vi "BioFeedback16(Intermittent Saving).vi"(7 "Frames Per Second":dbl=30.0, 9 "Start Trial":bool, 11 "End Trial":bool, 12 "Data Directory":path, 13 "File Name":string) -> ()   [LabVIEW 2016]
uses:
  customSubVIs/Control 1.ctl
  <vilib>/Waveform/WDTFileIO.llb/Export Waveforms To Spreadsheet File (1D).vi
  <vilib>/Utility/file.llb/Write Delimited Spreadsheet (DBL).vi
  <vilib>/Utility/file.llb/Write Delimited Spreadsheet (I64).vi
  <vilib>/Utility/error.llb/DialogType.ctl
panel:
  out "MVC Buffer Index":dbl=3.0
  in  "DisplayDataPath":path
  in  "FilteredDataPath":path
  in  "RawDataPath":path
  in  "MVC Number":dbl=1.0
  out "Save MVC":bool
  out "Display Buffer":dbl[][](array[numeric])
  out "Display Buffer Index":dbl=3.0
  out "FilteredTrialData Display Channel":waveform(dbl)(graph)
  out "Raw Trial Data Display Channel":waveform(dbl)(graph)
  out "EndProcessTic":u32
  out "StartProcessTic":u32
  out "EndRecordTic":u32
  out "startRecordTic":u32
  out "Start UI":timestamp
  out "UI Elapsed Time":u32
  out "End UI":timestamp
  out "End Process":timestamp
  out "Start Process":timestamp
  out "End Record":timestamp
  out "Start Record":timestamp
  out "Process Elapsed Time":u32
  out "Record Elapsed Time":u32
  out "FilteredTrialData":waveform(dbl)[](graph)
  out "FilteredAndRectified":waveform(dbl)[](graph) caption="Filtered and Rectified"
  out "FilteredDataArray":waveform(dbl)[](array[waveform])
  in  "DisplayChannel":dbl
  out "DisplayTrialData":T1
  out "DisplayValueByChannel":dbl[](array[numeric])
  out "MVCBufferSize":dbl
  in  "MVC Window Size (s)":dbl=0.5
  out "MVC Buffer":dbl[][](array[numeric])
  out "GetMaxStartTime":timestamp
  in  "SecondsToAcquireMax":dbl=10.0
  out "MVCArray":dbl[](array[numeric])
  out "RawTrialData":waveform(dbl)[](array[waveform])
  in  "UI Ampl Error Path":path=path "C:/Users/Tinggroup/Desktop/VRMuscleActivationVisualizer/VRBiofeedback_v2/assets/BiofeedbackAmplitudeError.txt"
  out "DisplayActivation":dbl
  out "Get MVC":bool
  in  "resetMax":bool
  in  "startGetMax":bool
  in  "Amplitude Error":dbl
  in  "UI Data Path":path=path "C:/Users/Tinggroup/Desktop/VRMuscleActivationVisualizer/VRBiofeedback_v2/assets/LeftEMGData.txt"
  in  "EMG Input Device\nProduct Type":string="USB-6009"
  out "DisplayBarActivation":dbl(slide) caption="Left" max=1.0 scale=0.0..100.0
  out "NormalizedSignal8":dbl[](graph)
  out "NormalizedSignal7":dbl[](graph)
  out "NormalizedSignal6":dbl[](graph)
  out "NormalizedSignal5":dbl[](graph)
  out "NormalizedSignal4":dbl[](graph)
  out "NormalizedSignal3":dbl[](graph)
  out "NormalizedSignal2":dbl[](graph)
  out "NormalizedSignal1":dbl[](graph)
  out "Raw Trial Data Wfm":waveform(dbl)[](graph)
  in  "UI Percent Path":path=path "C:/Users/Tinggroup/Desktop/VRMuscleActivationVisualizer/VRBiofeedback_v2/assets/BiofeedbackTargetPercentage.txt"
  in  "Target Percentage":dbl=10.0
  out "Trial In Progress":bool
  in  "Lower Cut-Off":dbl=20.0
  in  "Upper Cut-Off":dbl=300.0
  out "raw data":dynamicdata(graph)
  out "DisplayBufferSize":dbl
  out "Samples per frame":dbl
  out "Reset":bool=TRUE
  in  "Display Window Size (s)":dbl=0.5
  in  "Sample rate (Hz)":dbl=2000.0
  in  "End Program":bool
  # "Data To Be Saved (Not including Max Data)"
  # "Performance Metrics"
  # "Saving Trial Data"
  # "Small Window"
  # "Scale Max"
  # "Filter and Process Parameters"
  # "MVC Buffer"
  # "Set Target"
  # "Display Parameters"
  # "Changes are made instantly and cause moving average to reset to zero"
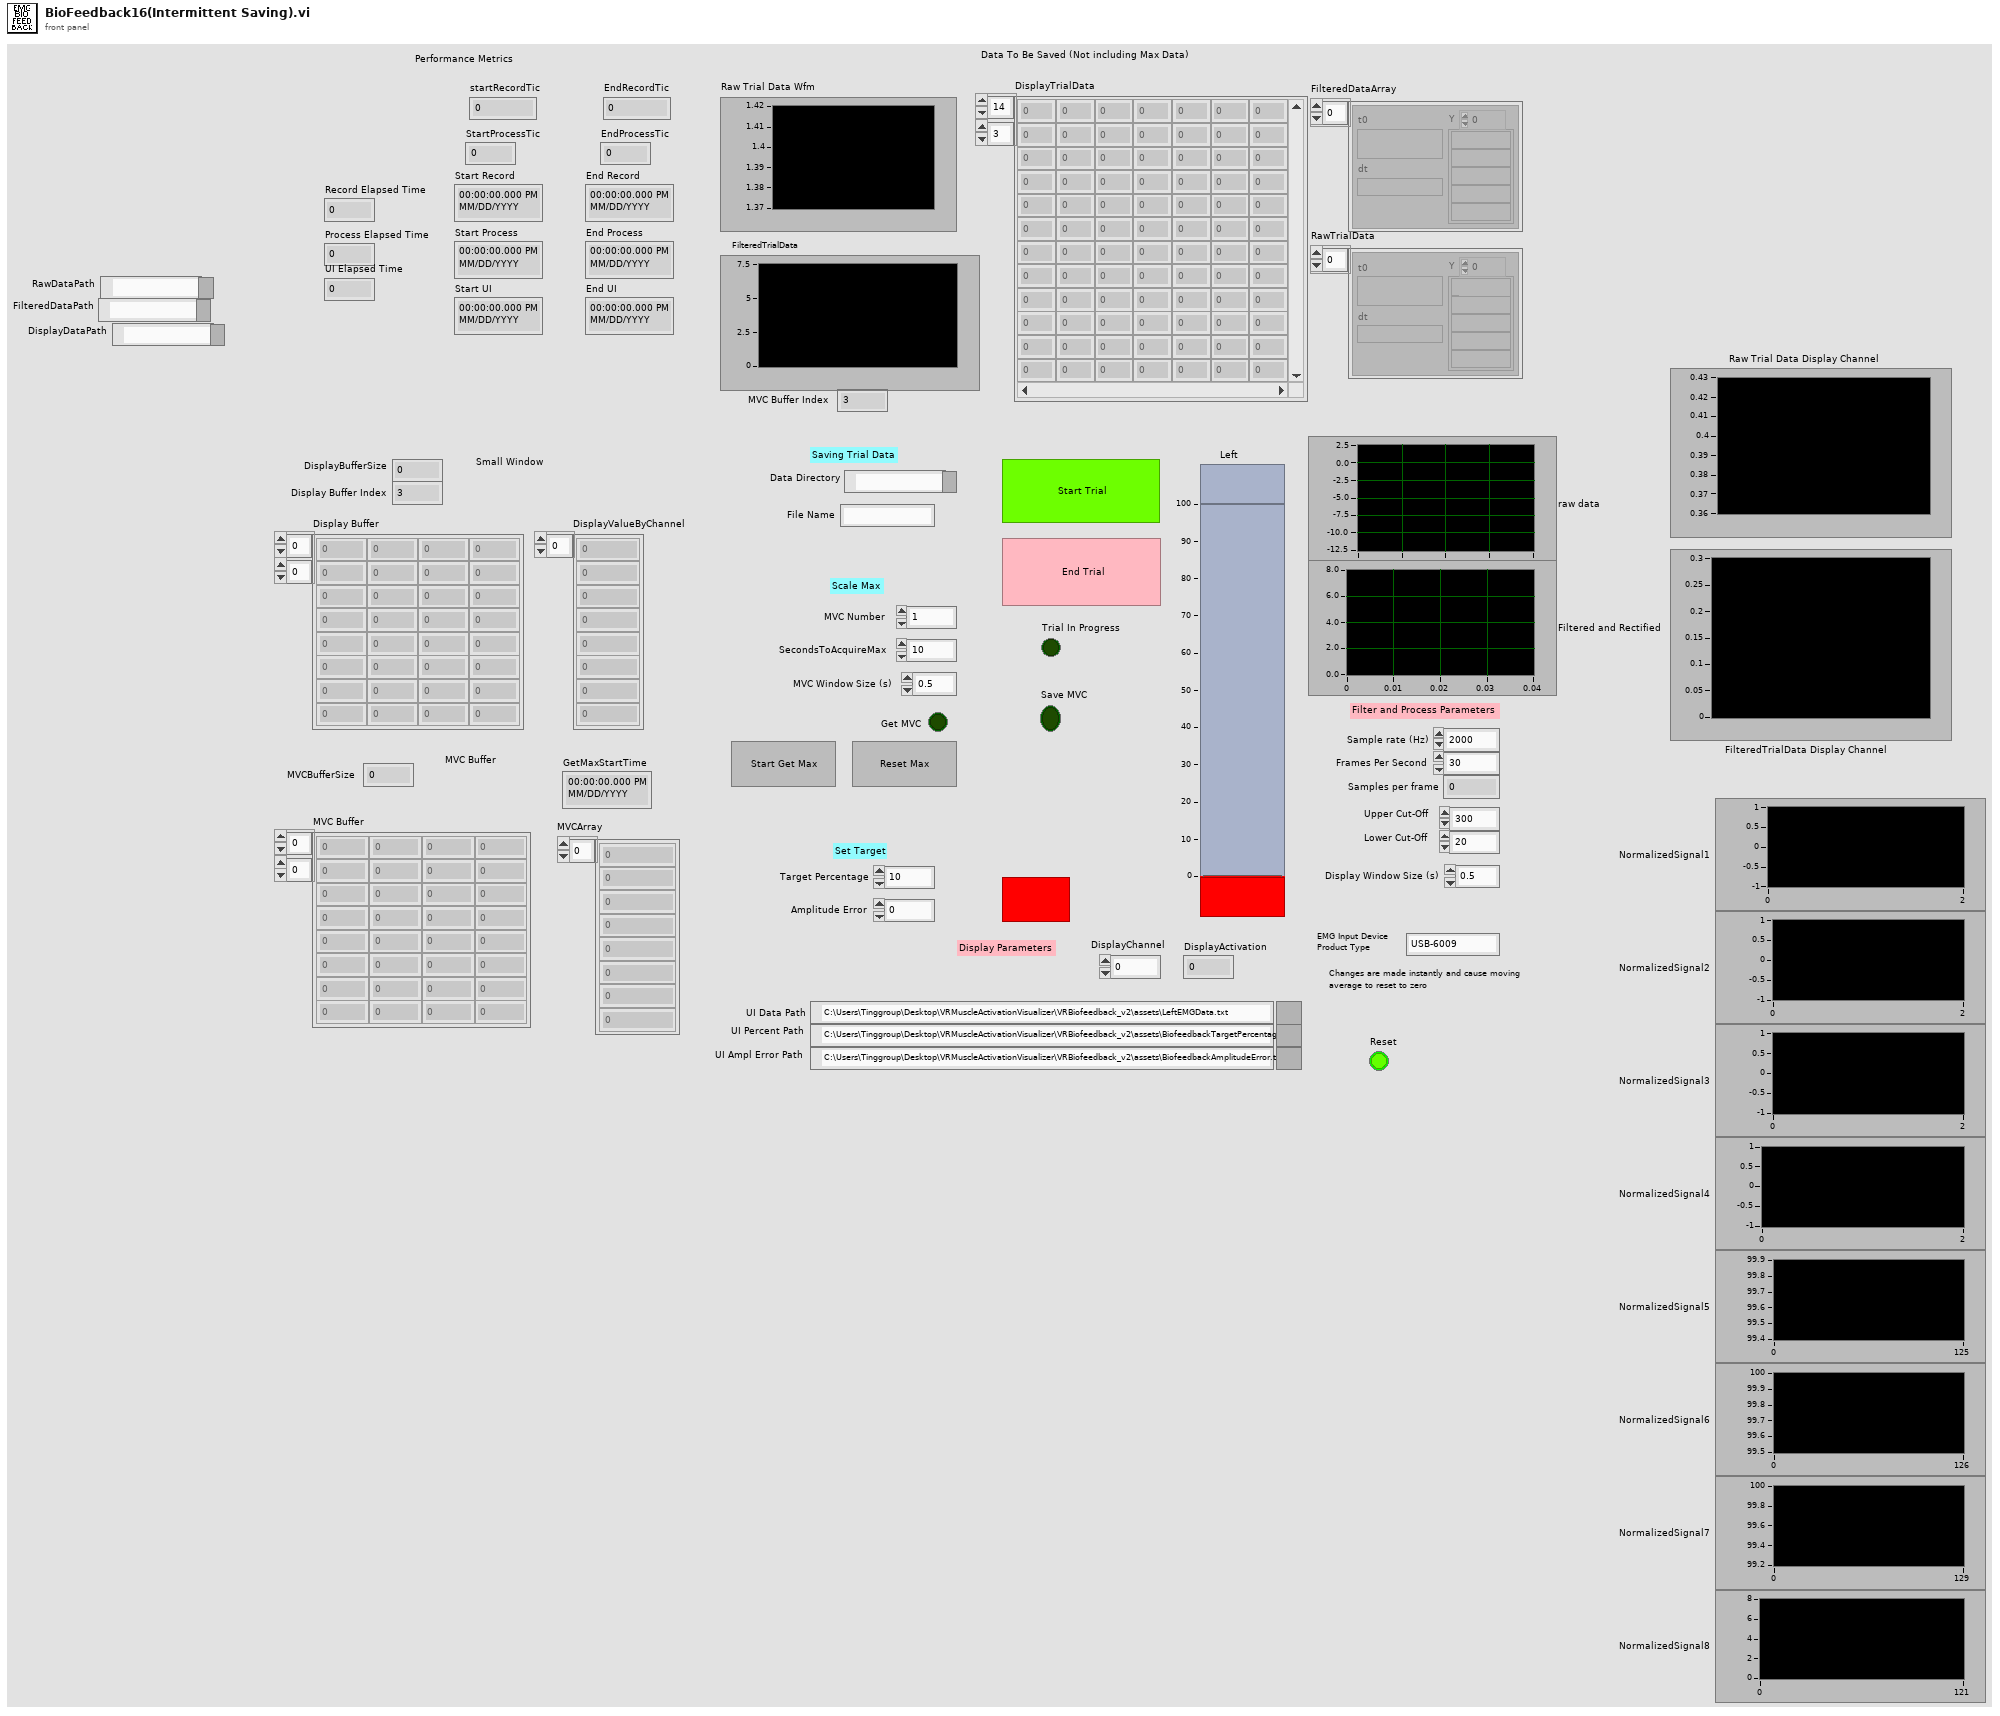
[diagram p1: front panel]
types:
  T1 = typedef "Control 1.ctl" = dbl[][]
  T2 = typedef "DialogType.ctl" = u16
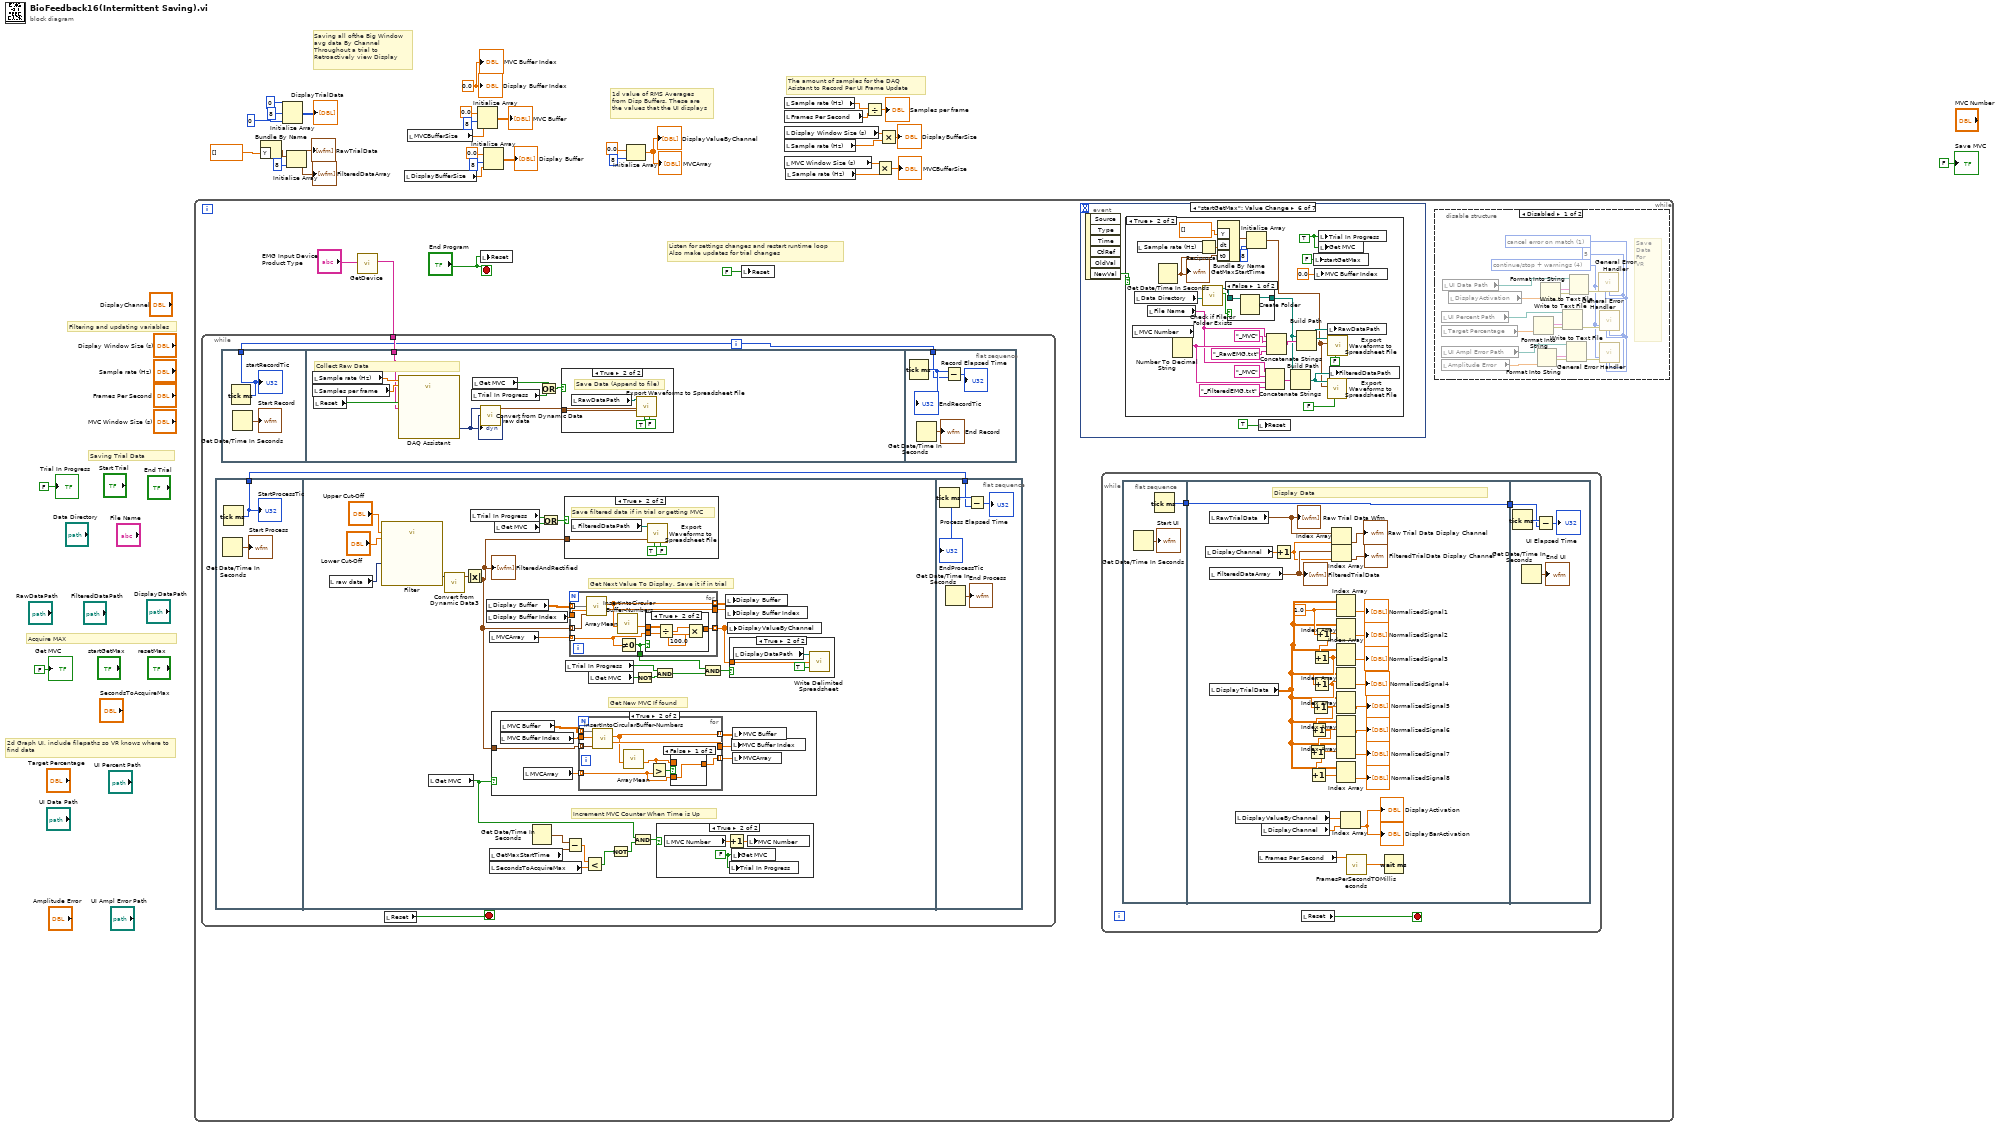
[diagram p0: block diagram]
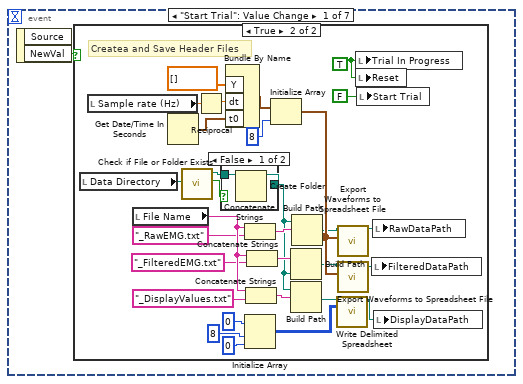
[diagram p3: hidden frame]
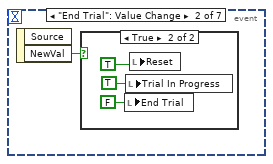
[diagram p6: hidden frame]
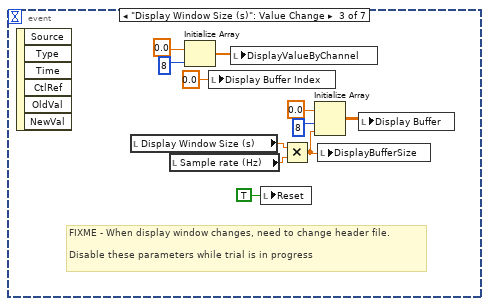
[diagram p8: hidden frame]
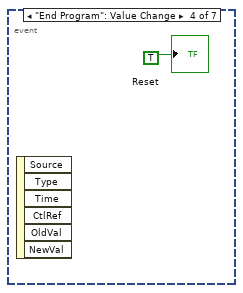
[diagram p9: hidden frame]
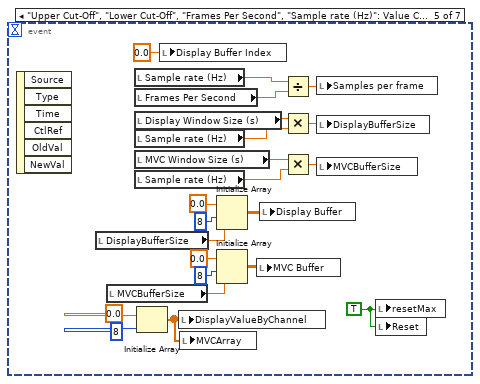
[diagram p10: hidden frame]
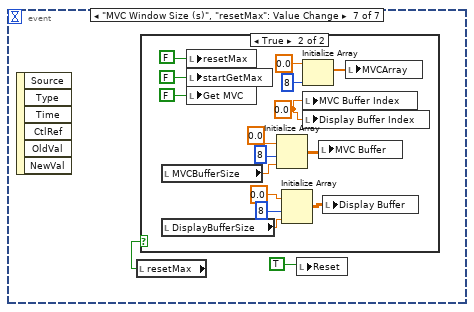
[diagram p13: hidden frame]
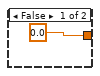
[diagram p19: hidden frame]
diagram:
  w1 = 0.0 ("Display Buffer Index")
  # "The amount of samples for the DAQ Asistant to Record Per UI Frame Update"
  # "Saving all ofthe Big Window \navg data By Channel\nThroughout a trial to \nRetroactively view Display"
  # "1d value of RMS Averages\nfrom Disp Buffers. These are\nthe values that the UI displays"
  # "Acquire MAX"
  # "Filtering and updating variables"
  # "Saving Trial Data"
  # "2d Graph UI, include filepaths so VR knows where to find data"
  n1 = while {
    stop <- "End Program" stop-if-true
    # "Listen for settings changes and restart runtime loop\nAlso make updates for trial changes"
    n2 = call "GetDevice.vi"("EMG Input Device\nProduct Type"="EMG Input Device\nProduct Type") -> ("DAQmx Device Name"=w35:tag)  [unwired: 10 in]
    n3 = while {
      tunnel: w35 -> [w214]
      stop <- w213 stop-if-true
      n4 = flat-sequence {
        tunnel: [w216] -> w212
        tunnel: w212 -> [w290]
        frame #0 {
          n5 = Get Date/Time In Seconds() -> (seconds since 1Jan1904=→"Start Process":timestamp)
          n6 = Tick Count (ms)() -> (millisecond timer value=w216:u32)
          "StartProcessTic" <- w216
        }
        frame #1 {
          # "Increment MVC Counter When Time is Up"
          # "Get New MVC If found"
          # "Get Next Value To Display, Save it if in trial"
          n7 = local read "raw data"() -> (w239:dynamicdata)
          n8 = call "Filter"("Lower Cut-Off"="Lower Cut-Off", "Upper Cut-Off"="Upper Cut-Off", "Signal"=w239) -> ("Filtered Signal"=w245:dynamicdata)  [unwired: 7 in, 1 out]
          n9 = local read "Get MVC"() -> (w223:bool)
          n10 = call "Convert from Dynamic Data3"("Dynamic Data Type"=w245) -> ("Array of Waveform"=w244:waveform(dbl)[])  [unwired: 3 in]
          n11 = Absolute Value(x=w244) -> (abs(x)=w228:waveform(dbl)[])
          "FilteredAndRectified" <- w228
          n12 = local read "Trial In Progress"() -> (w241:bool)
          n13 = local read "Display Buffer"() -> (w237:dbl[][])
          n14 = local read "Display Buffer Index"() -> (w236:dbl)
          n15 = local read "MVCArray"() -> (w233:dbl[])
          n16 = local read "GetMaxStartTime"() -> (w229:timestamp)
          n17 = local read "SecondsToAcquireMax"() -> (w232:dbl)
          n18 = case shown="True" w223 {
            tunnel: w228 -> [_ w256]
            frame False {
            }
            frame True {
              n19 = local read "MVC Buffer Index"() -> (w258:dbl)
              n20 = local read "MVC Buffer"() -> (w257:dbl[][])
              n21 = local read "MVCArray"() -> (w255:dbl[])
              n22 = for {
                tunnel: w257 -> [w267] mode=indexing
                tunnel: w258 -> [w259]
                tunnel: [w266] -> w252
                tunnel: w256 -> [w265] mode=indexing
                tunnel: w255 -> [w261] mode=indexing
                tunnel: [w260] -> w254 mode=indexing
                tunnel: [w262] -> w253 mode=indexing
                n23 = call "InsertIntoCircularBuffer-Numbers.vi"("NewElements"=w265, "StartIndex"=w259, "Buffer"=w267) -> ("New Start Index"=w266:dbl, "UpdatedBuffer"=w262:dbl[])  [unwired: 7 in]
                n24 = call "ArrayMean.vi"("Array"=w262) -> ("Mean"=w263:dbl)  [unwired: 10 in]
                n25 = Greater?(x=w263, y=w261) -> (0:w264:bool)
                n26 = case shown="False" w264 {
                  tunnel: w263 -> [_ w269]
                  tunnel: [w268 w269] -> w260
                  tunnel: w261 -> [w268 _]
                  frame False {
                  }
                  frame True {
                  }
                }
              }
              n27 = local write "MVC Buffer Index"(w252) -> ()
              n28 = local write "MVC Buffer"(w253) -> ()
              n29 = local write "MVCArray"(w254) -> ()
            }
          }
          n30 = local read "Get MVC"() -> (w238:bool)
          n31 = Get Date/Time In Seconds() -> (seconds since 1Jan1904=w230:timestamp)
          n32 = Or(x=w241, y=w238) -> (x .or. y?=w240:bool)
          n33 = case shown="True" w240 {
            tunnel: w228 -> [_ w285]
            frame False {
            }
            frame True {
              # "Save filtered data if in trial or getting MVC"
              n34 = local read "FilteredDataPath"() -> (w286:path)
              n35 = call-poly <vilib>:"Export Waveforms to Spreadsheet File.vi"("header? (write header:T)"=FALSE, "append to file? (new file:F)"=TRUE, "waveforms"=w285, "file path (dialog if empty)"=w286) -> ()  [unwired: 6 in, 2 out]
            }
          }
          n36 = local read "Trial In Progress"() -> (w218:bool)
          n37 = Subtract(x=w230, y=w229) -> (x-y=w231:dbl)
          n38 = for {
            tunnel: w237 -> [w278] mode=indexing
            tunnel: w228 -> [w271] mode=indexing
            tunnel: w236 -> [w277]
            tunnel: [w275] -> w235 mode=indexing
            tunnel: [w276] -> w234
            tunnel: w233 -> [w273] mode=indexing
            tunnel: [w272] -> w224 mode=indexing
            tunnel: [w270] -> w221
            n39 = call "InsertIntoCircularBuffer-Numbers.vi"("NewElements"=w271, "StartIndex"=w277, "Buffer"=w278) -> ("New Start Index"=w276:dbl, "UpdatedBuffer"=w275:dbl[])  [unwired: 7 in]
            n40 = call "ArrayMean.vi"("Array"=w275) -> ("Mean"=w274:dbl)  [unwired: 10 in]
            n41 = Not Equal To 0?(x=w273) -> (x != 0?=w270:bool)
            n42 = case shown="True" w270 {
              tunnel: w274 -> [_ w283]
              tunnel: w273 -> [_ w284]
              tunnel: [0.0 w282] -> w272
              frame False {
              }
              frame True {
                n43 = Divide(x=w283, y=w284) -> (x/y=w281:dbl)
                n44 = Multiply(x=w281, y=100.0) -> (x*y=w282:dbl)
              }
            }
          }
          n45 = Less?(x=w231, y=w232) -> (x < y?=w227:bool)
          n46 = local read "Get MVC"() -> (w220:bool)
          n47 = Not(x=w227) -> (.not. x?=w226:bool)
          n48 = And(x=w223, y=w226) -> (x .and. y?=w225:bool)
          n49 = Not(x=w220) -> (.not. x?=w219:bool)
          n50 = And(x=w218, y=w219) -> (x .and. y?=w217:bool)
          n51 = case shown="True" w225 {
            frame False {
            }
            frame True {
              w249 = FALSE ("Get MVC")
              n52 = local read "MVC Number"() -> (w250:dbl)
              n53 = Increment(x=w250) -> (x+1=w251:dbl)
              n54 = local write "Trial In Progress"(w249) -> ()
              n55 = local write "Get MVC"(w249) -> ()
              n56 = local write "MVC Number"(w251) -> ()
            }
          }
          n57 = And(x=w221, y=w217) -> (x .and. y?=w222:bool)
          n58 = local write "Display Buffer"(w235) -> ()
          n59 = local write "Display Buffer Index"(w234) -> ()
          n60 = local write "DisplayValueByChannel"(w224) -> ()
          n61 = case shown="True" w222 {
            tunnel: w224 -> [_ w247]
            frame False {
            }
            frame True {
              n62 = local read "DisplayDataPath"() -> (w246:path)
              n63 = call-poly <vilib>:"Write Delimited Spreadsheet.vi"("file path (dialog if empty)"=w246, "1D data"=w247, "append to file? (new file:F)"=TRUE) -> ()  [unwired: 11 in, 2 out]
            }
          }
        }
        frame #2 {
          n64 = Tick Count (ms)() -> (millisecond timer value=w291:u32)
          "EndProcessTic" <- w291
          n65 = Get Date/Time In Seconds() -> (seconds since 1Jan1904=→"End Process":timestamp)
          n66 = Subtract(x=w291, y=w290) -> (x-y=→"Process Elapsed Time":u32)
        }
      }
      n67 = flat-sequence {
        tunnel: [w294] -> w211
        tunnel: w214 -> [w299]
        tunnel: w211 -> [w308]
        frame #0 {
          n68 = Tick Count (ms)() -> (millisecond timer value=w294:u32)
          "startRecordTic" <- w294
          n69 = Get Date/Time In Seconds() -> (seconds since 1Jan1904=→"Start Record":timestamp)
        }
        frame #1 {
          # "Collect Raw Data"
          n70 = local read "Sample rate (Hz)"() -> (w302:dbl)
          n71 = local read "Samples per frame"() -> (w301:dbl)
          n72 = local read "Reset"() -> (w300:bool)
          n73 = call "DAQ Assistant"("rate"=w302, "number of samples"=w301, "stop (T)"=w300, "device name"=w299) -> ("data"=w296:dynamicdata)  [unwired: 13 in, 2 out]
          "raw data" <- w296
          n74 = local read "Trial In Progress"() -> (w298:bool)
          n75 = local read "Get MVC"() -> (w297:bool)
          n76 = call "Convert from Dynamic Data"("Dynamic Data Type"=w296) -> ("Array of Waveform"=w303:waveform(dbl)[])  [unwired: 3 in]
          n77 = Or(x=w297, y=w298) -> (x .or. y?=w295:bool)
          n78 = case shown="True" w295 {
            tunnel: w303 -> [_ w305]
            frame False {
            }
            frame True {
              # "Save Data (Append to file)"
              n79 = local read "RawDataPath"() -> (w304:path)
              n80 = call-poly <vilib>:"Export Waveforms to Spreadsheet File.vi"("header? (write header:T)"=FALSE, "append to file? (new file:F)"=TRUE, "waveforms"=w305, "file path (dialog if empty)"=w304) -> ()  [unwired: 6 in, 2 out]
            }
          }
        }
        frame #2 {
          n81 = Tick Count (ms)() -> (millisecond timer value=w309:u32)
          "EndRecordTic" <- w309
          n82 = Get Date/Time In Seconds() -> (seconds since 1Jan1904=→"End Record":timestamp)
          n83 = Subtract(x=w309, y=w308) -> (x-y=→"Record Elapsed Time":u32)
        }
      }
      n84 = local read "Reset"() -> (w213:bool)
    }
    n85 = local write "Reset"("End Program") -> ()
    n86 = local write "Reset"(FALSE) -> ()
    n87 = event shown="[5] \"startGetMax\": Value Change" {
      selector: _ -> [_ _ _ _ _ _ _]
      dyn-events: _ -> [_ _ _ _ _ _ _]
      timeout: _ -> [_ _ _ _ _ _ _]
      event "Start Trial": Value Change {
        n88 = event-data() -> ("NewVal"=w93:bool)  [unwired: 1 in, 1 out]
        n89 = case shown="True" w93 {
          frame False {
          }
          frame True {
            w120 = TRUE ("Trial In Progress")
            # "Createa and Save Header Files"
            n90 = local read "Data Directory"() -> (w107:path)
            n91 = local read "Sample rate (Hz)"() -> (w116:dbl)
            n92 = local read "File Name"() -> (w113:string)
            n93 = Get Date/Time In Seconds() -> (seconds since 1Jan1904=w114:timestamp)
            n94 = call <vilib>:"Check if File or Folder Exists.vi"("path"=w107) -> ("file or folder exists?"=w106:bool, "dup path"=w105:path)  [unwired: 8 in, 1 out]
            n95 = Reciprocal(x=w116) -> (1/x=w115:dbl)
            n96 = case shown="False" w106 {
              tunnel: [w121 w123] -> w104
              tunnel: w105 -> [w122 w123]
              frame False {
                n97 = Create Folder(path (use dialog)=w122) -> (created path=w121:path)  [unwired: 2 in, 2 out]
              }
              frame True {
              }
            }
            n98 = Bundle By Name("Y"=dbl[] [], "dt"=w115, "t0"=w114) -> (w119:waveform(dbl))  [unwired: 1 in]
            n99 = Concatenate Strings(w113, "_RawEMG.txt" ("string")) -> (w108:string)
            n100 = Initialize Array(0, 8 ("dimension size"), 0 ("dimension size")) -> (w95:i32[][])
            n101 = Concatenate Strings(w113, "_DisplayValues.txt" ("string")) -> (w111:string)
            n102 = Concatenate Strings(w113, "_FilteredEMG.txt" ("string")) -> (w109:string)
            n103 = Initialize Array(w119, 8 ("dimension size")) -> (w103:waveform(dbl)[])
            n104 = Build Path(base path=w104, name or relative path=w109) -> (appended path=w100:path)
            n105 = Build Path(base path=w104, name or relative path=w111) -> (appended path=w99:path)
            n106 = Build Path(base path=w104, name or relative path=w108) -> (appended path=w101:path)
            n107 = call-poly <vilib>:"Write Delimited Spreadsheet.vi"("file path (dialog if empty)"=w99, "2D data"=w95) -> ()  [unwired: 12 in, 2 out]
            n108 = call-poly <vilib>:"Export Waveforms to Spreadsheet File.vi"("waveforms"=w103, "file path (dialog if empty)"=w101) -> ()  [unwired: 8 in, 2 out]
            n109 = call-poly <vilib>:"Export Waveforms to Spreadsheet File.vi"("waveforms"=w103, "file path (dialog if empty)"=w100) -> ()  [unwired: 8 in, 2 out]
            n110 = local write "Trial In Progress"(w120) -> ()
            n111 = local write "Reset"(w120) -> ()
            n112 = local write "Start Trial"(FALSE ("Start Trial")) -> ()
            n113 = local write "FilteredDataPath"(w100) -> ()
            n114 = local write "RawDataPath"(w101) -> ()
            n115 = local write "DisplayDataPath"(w99) -> ()
          }
        }
      }
      event "End Trial": Value Change {
        n116 = event-data() -> ("NewVal"=w124:bool)  [unwired: 1 in, 1 out]
        n117 = case shown="True" w124 {
          frame False {
          }
          frame True {
            n118 = local write "End Trial"(FALSE ("End Trial")) -> ()
            n119 = local write "Trial In Progress"(TRUE ("Trial In Progress")) -> ()
            n120 = local write "Reset"(TRUE ("Reset Data Acquisition\nAnd UI Updating")) -> ()
          }
        }
      }
      event "Display Window Size (s)": Value Change {
        # "FIXME - When display window changes, need to change header file.\n\nDisable these parameters while trial is in progress"
        n121 = event-data() -> ()  [unwired: 1 in, 6 out]
        n122 = local read "Display Window Size (s)"() -> (w130:dbl)
        n123 = local read "Sample rate (Hz)"() -> (w129:dbl)
        n124 = Initialize Array(0.0 ("element"), 8 ("dimension size")) -> (w135:dbl[])
        n125 = local write "Display Buffer Index"(0.0 ("Display Buffer Index")) -> ()
        n126 = local write "DisplayValueByChannel"(w135) -> ()
        n127 = local write "Reset"(TRUE ("Reset")) -> ()
        n128 = Multiply(x=w130, y=w129) -> (x*y=w128:dbl)
        n129 = Initialize Array(0.0 ("element"), 8 ("dimension size"), w128) -> (w131:dbl[][])
        n130 = local write "DisplayBufferSize"(w128) -> ()
        n131 = local write "Display Buffer"(w131) -> ()
      }
      event "End Program": Value Change {
        n132 = event-data() -> ()  [unwired: 1 in, 6 out]
        "Reset" <- TRUE
      }
      event "Upper Cut-Off", "Lower Cut-Off", "Frames Per Second", "Sample rate (Hz)": Value Change {
        w146 = TRUE
        n133 = event-data() -> ()  [unwired: 1 in, 6 out]
        n134 = local read "DisplayBufferSize"() -> (w151:dbl)
        n135 = local read "MVCBufferSize"() -> (w143:dbl)
        n136 = local read "Sample rate (Hz)"() -> (w161:dbl)
        n137 = local read "Frames Per Second"() -> (w160:dbl)
        n138 = local read "Display Window Size (s)"() -> (w158:dbl)
        n139 = local read "Sample rate (Hz)"() -> (w157:dbl)
        n140 = local read "MVC Window Size (s)"() -> (w156:dbl)
        n141 = local read "Sample rate (Hz)"() -> (w155:dbl)
        n142 = Initialize Array(0.0 ("element"), 8 ("dimension size")) -> (w145:dbl[])
        n143 = local write "Display Buffer Index"(0.0 ("Display Buffer Index")) -> ()
        n144 = local write "DisplayValueByChannel"(w145) -> ()
        n145 = local write "MVCArray"(w145) -> ()
        n146 = Initialize Array(0.0 ("element"), 8 ("dimension size"), w151) -> (w149:dbl[][])
        n147 = Initialize Array(0.0 ("element"), 8 ("dimension size"), w143) -> (w141:dbl[][])
        n148 = local write "MVC Buffer"(w141) -> ()
        n149 = local write "Display Buffer"(w149) -> ()
        n150 = Divide(x=w161, y=w160) -> (x/y=w159:dbl)
        n151 = Multiply(x=w158, y=w157) -> (x*y=w153:dbl)
        n152 = Multiply(x=w156, y=w155) -> (x*y=w154:dbl)
        n153 = local write "Samples per frame"(w159) -> ()
        n154 = local write "DisplayBufferSize"(w153) -> ()
        n155 = local write "MVCBufferSize"(w154) -> ()
        n156 = local write "resetMax"(w146) -> ()
        n157 = local write "Reset"(w146) -> ()
      }
      event "startGetMax": Value Change {
        n158 = event-data() -> ("NewVal"=w163:bool)  [unwired: 1 in, 5 out]
        n159 = case shown="True" w163 {
          frame False {
          }
          frame True {
            w168 = TRUE ("Trial In Progress")
            n160 = local read "MVC Number"() -> (w182:dbl)
            n161 = local read "Data Directory"() -> (w186:path)
            n162 = local read "Sample rate (Hz)"() -> (w178:dbl)
            n163 = local read "File Name"() -> (w175:string)
            n164 = Get Date/Time In Seconds() -> (seconds since 1Jan1904=w176:timestamp)
            "GetMaxStartTime" <- w176
            n165 = Number To Decimal String(number=w182) -> (decimal integer string=w185:string)  [unwired: 1 in]
            n166 = Reciprocal(x=w178) -> (1/x=w177:dbl)
            n167 = call <vilib>:"Check if File or Folder Exists.vi"("path"=w186) -> ("file or folder exists?"=w183:bool, "dup path"=w190:path)  [unwired: 8 in, 1 out]
            n168 = Bundle By Name("Y"=dbl[] [], "dt"=w177, "t0"=w176) -> (w180:waveform(dbl))  [unwired: 1 in]
            n169 = case shown="False" w183 {
              tunnel: w190 -> [w192 w193]
              tunnel: [w191 w193] -> w172
              frame False {
                n170 = Create Folder(path (use dialog)=w192) -> (created path=w191:path)  [unwired: 2 in, 2 out]
              }
              frame True {
              }
            }
            n171 = Initialize Array(w180, 8 ("dimension size")) -> (w167:waveform(dbl)[])
            n172 = Concatenate Strings(w175, "_MVC" ("string"), w185, "_FilteredEMG.txt" ("string")) -> (w188:string)
            n173 = Concatenate Strings(w175, "_MVC" ("string"), w185, "_RawEMG.txt" ("string")) -> (w187:string)
            n174 = Build Path(base path=w172, name or relative path=w188) -> (appended path=w170:path)
            n175 = Build Path(base path=w172, name or relative path=w187) -> (appended path=w181:path)
            n176 = local write "startGetMax"(FALSE ("Start Trial")) -> ()
            n177 = local write "MVC Buffer Index"(0.0 ("MVC Buffer Indes")) -> ()
            n178 = local write "Trial In Progress"(w168) -> ()
            n179 = local write "Get MVC"(w168) -> ()
            n180 = local write "RawDataPath"(w181) -> ()
            n181 = call-poly <vilib>:"Export Waveforms to Spreadsheet File.vi"("append to file? (new file:F)"=FALSE, "waveforms"=w167, "file path (dialog if empty)"=w170) -> ()  [unwired: 7 in, 2 out]
            n182 = call-poly <vilib>:"Export Waveforms to Spreadsheet File.vi"("append to file? (new file:F)"=FALSE, "waveforms"=w167, "file path (dialog if empty)"=w181) -> ()  [unwired: 7 in, 2 out]
            n183 = local write "FilteredDataPath"(w170) -> ()
          }
        }
        n184 = local write "Reset"(TRUE ("Reset Data Acquisition\nAnd UI Updating")) -> ()
      }
      event "MVC Window Size (s)", "resetMax": Value Change {
        n185 = event-data() -> ()  [unwired: 1 in, 6 out]
        n186 = local read "resetMax"() -> (w194:bool)
        n187 = case shown="True" w194 {
          frame False {
          }
          frame True {
            w196 = 0.0 ("MVC Buffer Index")
            n188 = local read "MVCBufferSize"() -> (w202:dbl)
            n189 = local read "DisplayBufferSize"() -> (w198:dbl)
            n190 = local write "resetMax"(FALSE ("endGetMax")) -> ()
            n191 = local write "startGetMax"(FALSE ("startGetMax")) -> ()
            n192 = local write "Get MVC"(FALSE ("Acquiring Max")) -> ()
            n193 = Initialize Array(0.0 ("element"), 8 ("dimension size"), w202) -> (w201:dbl[][])
            n194 = Initialize Array(0.0 ("element"), 8 ("dimension size"), w198) -> (w197:dbl[][])
            n195 = Initialize Array(0.0 ("element"), 8 ("dimension size")) -> (w205:dbl[])
            n196 = local write "MVC Buffer Index"(w196) -> ()
            n197 = local write "Display Buffer Index"(w196) -> ()
            n198 = local write "MVC Buffer"(w201) -> ()
            n199 = local write "Display Buffer"(w197) -> ()
            n200 = local write "MVCArray"(w205) -> ()
          }
        }
        n201 = local write "Reset"(TRUE ("Reset Data Acquisition\nAnd UI Updating")) -> ()
      }
    }
    n202 = while {
      stop <- w55 stop-if-true
      n203 = flat-sequence {
        tunnel: [w59] -> w57
        tunnel: [w88] -> w56
        tunnel: w57 -> [w88]
        tunnel: w56 -> [w89]
        frame #0 {
          n204 = Get Date/Time In Seconds() -> (seconds since 1Jan1904=→"Start UI":timestamp)
          n205 = Tick Count (ms)() -> (millisecond timer value=w59:u32)
        }
        frame #1 {
          w62 = 1.0 ("x")
          # "Display Data"
          n206 = local read "DisplayChannel"() -> (w83:dbl)
          n207 = local read "RawTrialData"() -> (w78:waveform(dbl)[])
          "Raw Trial Data Wfm" <- w78
          n208 = local read "DisplayTrialData"() -> (w61:T1)
          n209 = local read "FilteredDataArray"() -> (w82:waveform(dbl)[])
          "FilteredTrialData" <- w82
          n210 = local read "DisplayValueByChannel"() -> (w87:dbl[])
          n211 = local read "Frames Per Second"() -> (w85:dbl)
          n212 = local read "DisplayChannel"() -> (w84:dbl)
          n213 = Increment(x=w83) -> (x+1=w81:dbl)
          n214 = Increment(x=w62) -> (x+1=w63:dbl)
          n215 = Increment(x=w63) -> (x+1=w64:dbl)
          n216 = Increment(x=w64) -> (x+1=w65:dbl)
          n217 = Increment(x=w65) -> (x+1=w66:dbl)
          n218 = Increment(x=w66) -> (x+1=w67:dbl)
          n219 = Increment(x=w67) -> (x+1=w68:dbl)
          n220 = Increment(x=w68) -> (x+1=w69:dbl)
          n221 = Index Array(array=w78, index=w81) -> (element=→"Raw Trial Data Display Channel":waveform(dbl))
          n222 = Index Array(array=w82, index=w81) -> (element=→"FilteredTrialData Display Channel":waveform(dbl))
          n223 = Index Array(array=w61, index (row)=w62) -> (element=→"NormalizedSignal1":dbl[])  [unwired: 1 in]
          n224 = Index Array(array=w61, index (row)=w63) -> (element=→"NormalizedSignal2":dbl[])  [unwired: 1 in]
          n225 = Index Array(array=w61, index (row)=w64) -> (element=→"NormalizedSignal3":dbl[])  [unwired: 1 in]
          n226 = Index Array(array=w61, index (row)=w65) -> (element=→"NormalizedSignal4":dbl[])  [unwired: 1 in]
          n227 = Index Array(array=w61, index (row)=w66) -> (element=→"NormalizedSignal5":dbl[])  [unwired: 1 in]
          n228 = Index Array(array=w61, index (row)=w67) -> (element=→"NormalizedSignal6":dbl[])  [unwired: 1 in]
          n229 = Index Array(array=w61, index (row)=w68) -> (element=→"NormalizedSignal7":dbl[])  [unwired: 1 in]
          n230 = Index Array(array=w61, index (row)=w69) -> (element=→"NormalizedSignal8":dbl[])  [unwired: 1 in]
          n231 = Index Array(array=w87, index=w84) -> (element=→"DisplayBarActivation" →"DisplayActivation":dbl)
          n232 = call "FramesPerSecondTOMilliseconds.vi"("Thermometer\nFps"=w85) -> ("x*y"=w86:dbl)  [unwired: 10 in]
          n233 = Wait (ms)(milliseconds to wait=w86) -> ()  [unwired: 1 out]
        }
        frame #2 {
          n234 = Tick Count (ms)() -> (millisecond timer value=w90:u32)
          n235 = Get Date/Time In Seconds() -> (seconds since 1Jan1904=→"End UI":timestamp)
          n236 = Subtract(x=w90, y=w89) -> (x-y=→"UI Elapsed Time":u32)
        }
      }
      n237 = local read "Reset"() -> (w55:bool)
    }
    n238 = disable-structure shown="Disabled" {
      frame Disabled {
        w39 = T2 4 items=["no dialog", "OK message", "continue or stop message", "OK message + warnings", "continue/stop + warnings"] ("type of dialog (OK msg:1)")
        w38 = 1 items=["no exception", "cancel error on match", "set error on match"] ("[exception action] (none:0)")
        w37 = 5 ("[exception code]")
        # "Save\nData\nFor\nVR"
        n239 = local read "UI Ampl Error Path"() -> (w40:path)
        n240 = local read "Amplitude Error"() -> (w41:dbl)
        n241 = local read "UI Percent Path"() -> (w46:path)
        n242 = local read "Target Percentage"() -> (w45:dbl)
        n243 = local read "UI Data Path"() -> (w52:path)
        n244 = local read "DisplayActivation"() -> (w50:dbl)
        n245 = Format Into String(w45) -> (resulting string=w47:string, error out=w48:errorcluster)  [unwired: 3 in]
        n246 = Format Into String(w41) -> (resulting string=w42:string, error out=w43:errorcluster)  [unwired: 3 in]
        n247 = Format Into String(w50) -> (resulting string=w51:string, error out=w53:errorcluster)  [unwired: 3 in]
        n248 = Write to Text File(file (use dialog)=w46, text=w47, error in=w48) -> (error out=w49:errorcluster)  [unwired: 1 in, 2 out]
        n249 = Write to Text File(file (use dialog)=w40, text=w42, error in=w43) -> (error out=w44:errorcluster)  [unwired: 1 in, 2 out]
        n250 = Write to Text File(file (use dialog)=w52, text=w51, error in=w53) -> (error out=w54:errorcluster)  [unwired: 1 in, 2 out]
        n251 = call <vilib>:"General Error Handler.vi"("type of dialog (OK msg:1)"=w39, "error in (no error)"=w54, "[exception action] (none:0)"=w38, "[exception code]"=w37) -> ()  [unwired: 7 in, 5 out]
        n252 = call <vilib>:"General Error Handler.vi"("type of dialog (OK msg:1)"=w39, "error in (no error)"=w49, "[exception action] (none:0)"=w38, "[exception code]"=w37) -> ()  [unwired: 7 in, 5 out]
        n253 = call <vilib>:"General Error Handler.vi"("type of dialog (OK msg:1)"=w39, "error in (no error)"=w44, "[exception action] (none:0)"=w38, "[exception code]"=w37) -> ()  [unwired: 7 in, 5 out]
      }
      frame Enabled {
      }
    }
  }
  n254 = Bundle By Name("Y"=dbl[] []) -> (w24:waveform(dbl))  [unwired: 1 in]
  n255 = Initialize Array(0, 8 ("dimension size"), 0 ("dimension size")) -> (→"DisplayTrialData":i32[][])
  n256 = Initialize Array(w24, 8 ("dimension size")) -> (→"RawTrialData" →"FilteredDataArray":waveform(dbl)[])
  n257 = local read "DisplayBufferSize"() -> (w16:dbl)
  n258 = local read "MVCBufferSize"() -> (w29:dbl)
  n259 = Initialize Array(0.0 ("element"), 8 ("dimension size"), w29) -> (→"MVC Buffer":dbl[][])
  n260 = Initialize Array(0.0 ("element"), 8 ("dimension size"), w16) -> (→"Display Buffer":dbl[][])
  n261 = Initialize Array(0.0 ("element"), 8 ("dimension size")) -> (→"MVCArray" →"DisplayValueByChannel":dbl[])
  n262 = local read "Sample rate (Hz)"() -> (w4:dbl)
  n263 = local read "Frames Per Second"() -> (w5:dbl)
  n264 = local read "Display Window Size (s)"() -> (w8:dbl)
  n265 = local read "Sample rate (Hz)"() -> (w7:dbl)
  n266 = local read "MVC Window Size (s)"() -> (w10:dbl)
  n267 = local read "Sample rate (Hz)"() -> (w12:dbl)
  n268 = Divide(x=w4, y=w5) -> (x/y=→"Samples per frame":dbl)
  n269 = Multiply(x=w10, y=w12) -> (x*y=→"MVCBufferSize":dbl)
  n270 = Multiply(x=w8, y=w7) -> (x*y=→"DisplayBufferSize":dbl)
  "Trial In Progress" <- FALSE ("Trial In Progress")
  "Get MVC" <- FALSE ("Acquiring Max")
  "Display Buffer Index" <- w1
  "Save MVC" <- FALSE ("Saving")
  "MVC Buffer Index" <- w1
